vi "画色块.vi"(7 "位置":cluster{"x":i16, "y":i16}, 8 "块大小":cluster{"x":dbl, "y":dbl}, 9 "ID":string, 10 "颜色":u32(colorbox), 11 "picture in":picture) -> (3 "picture out":picture)   [LabVIEW 2016]
uses:
  <vilib>/picture/picture.llb/Draw True-Color Pixmap.vi
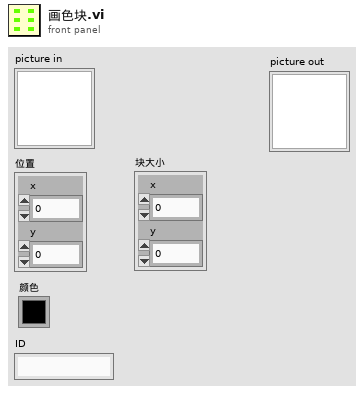
[diagram p1: front panel]
types:
  T1 = cluster{"horizontal":enum16{"left", "center", "right"}, "vertical":enum16{"top", "center", "bottom"}}
  T2 = cluster{"Width":i16, "Style":enum32{"Solid", "Dash", "Dot", "DashDot", "DashDotDot"}}
  T3 = cluster{"left":i16, "top":i16, "right":i16, "bottom":i16}
  T4 = typedef "imagedata.ctl" = cluster{"image type":i32, "image depth":i32, "image":u8[], "mask":u8[], "colors":u32[], "Rectangle":cluster{"left":i16, "top":i16, "right":i16, "bottom":i16}}
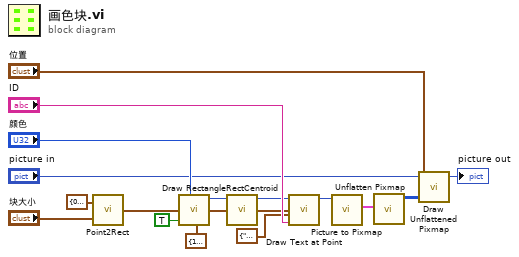
[diagram p0: block diagram]
diagram:
  n1 = call <vilib>:"Point2Rect.vi"("point b"="块大小", "point a"=cluster{"x":dbl, "y":dbl} {"x"=0.0, "y"=0.0}) -> ("rect"=w2:T3)
  n2 = call <vilib>:"Draw Rectangle.vi"("rect"=w2, "fill?(F)"=TRUE, "color(black)"="颜色", "pen"=T2 {"Width"=1, "Style"=enum."Solid"}) -> ("new picture"=w4:picture)  [unwired: 5 in]
  n3 = call <vilib>:"RectCentroid.vi"("rect"=w2) -> ("point"=w6:cluster{"x":i16, "y":i16})
  n4 = call <vilib>:"Draw Text at Point.vi"("text"="ID", "alignment(left, top)"=T1 {"horizontal"=enum."center", "vertical"=enum."center"}, "origin"=w6, "picture"=w4) -> ("new picture"=w9:picture)  [unwired: 6 in, 1 out]
  n5 = call <vilib>:"Picture to Pixmap.vi"("picture"=w9) -> ("image data"=w10:T4)  [unwired: 9 in, 1 out]
  n6 = call <vilib>:"Unflatten Pixmap.vi"("image data"=w10) -> ("24-bit pixmap"=w11:u32[][])  [unwired: 4 in, 6 out]
  n7 = call-poly <vilib>:"Draw Unflattened Pixmap.vi"("picture"="picture in", "top left point(0, 0)"="位置", "data (RGB format)"=w11) -> ("new picture"=→"picture out":picture)  [unwired: 6 in]
